vi "New Project.vi"(9 "DBSet":T1={"Server"="172.20.23.107", "DB"="HTPSDB", "PSW"="data'songyy", "User"="sa"}, 10 "UserID":string="L043460", 11 "厂区":string="清溪") -> ()   [LabVIEW 2011] (continued)
\n7714787500.000000#-39.000000#-4.400000#-18.000000#-10.000000#-3.000000#-30.000000#-30.000000\r\n7721031250.000000#-39.000000#-4.400000#-18.000000#-10.000000#-3.000000#-30.000000#-30.000000\r\n7727275000.000000#-39.000000#-4.400000#-18.000000#-10.000000#-3.000000#-30.000000#-30.000000\r\n7733518750.000000#-39.000000#-4.400000#-18.000000#-10.000000#-3.000000#-30.000000#-30.000000\r\n7739762500.000000#-39.000000#-4.400000#-18.000000#-10.000000#-3.000000#-30.000000#-30.000000\r\n7746006250.000000#-39.000000#-4.400000#-18.000000#-10.000000#-3.000000#-30.000000#-30.000000\r\n7752250000.000000#-39.000000#-4.400000#-18.000000#-10.000000#-3.000000#-30.000000#-30.000000\r\n7758493750.000000#-39.000000#-4.400000#-18.000000#-10.000000#-3.000000#-30.000000#-30.000000\r\n7764737500.000000#-39.000000#-4.400000#-18.000000#-10.000000#-3.000000#-30.000000#-30.000000\r\n7770981250.000000#-39.000000#-4.400000#-18.000000#-10.000000#-3.000000#-30.000000#-30.000000\r\n7777225000.000000#-39.000000#-4.400000#-18.000000#-10.000000#-3.000000#-30.000000#-30.000000\r\n7783468750.000000#-39.000000#-4.400000#-18.000000#-10.000000#-3.000000#-30.000000#-30.000000\r\n7789712500.000000#-39.000000#-4.400000#-18.000000#-10.000000#-3.000000#-30.000000#-30.000000\r\n7795956250.000000#-39.000000#-4.400000#-18.000000#-10.000000#-3.000000#-30.000000#-30.000000\r\n7802200000.000000#-39.000000#-4.400000#-18.000000#-10.000000#-3.000000#-30.000000#-30.000000\r\n7808443750.000000#-39.000000#-4.400000#-18.000000#-10.000000#-3.000000#-30.000000#-30.000000\r\n7814687500.000000#-39.000000#-4.400000#-18.000000#-10.000000#-3.000000#-30.000000#-30.000000\r\n7820931250.000000#-39.000000#-4.400000#-18.000000#-10.000000#-3.000000#-30.000000#-30.000000\r\n7827175000.000000#-39.000000#-4.400000#-18.000000#-10.000000#-3.000000#-30.000000#-30.000000\r\n7833418750.000000#-39.000000#-4.400000#-18.000000#-10.000000#-3.000000#-30.000000#-30.000000\r\n7839662500.000000#-39.000000#-4.400000#-18.000000#-10.000000#-3.000000#-30.000000#-30.000000\r\n7845906250.000000#-39.000000#-4.400000#-18.000000#-10.000000#-3.000000#-30.000000#-30.000000\r\n7852150000.000000#-39.000000#-4.400000#-18.000000#-10.000000#-3.000000#-30.000000#-30.000000\r\n7858393750.000000#-39.000000#-4.400000#-18.000000#-10.000000#-3.000000#-30.000000#-30.000000\r\n7864637500.000000#-39.000000#-4.400000#-18.000000#-10.000000#-3.000000#-30.000000#-30.000000\r\n7870881250.000000#-39.000000#-4.400000#-18.000000#-10.000000#-3.000000#-30.000000#-30.000000\r\n7877125000.000000#-39.000000#-4.400000#-18.000000#-10.000000#-3.000000#-30.000000#-30.000000\r\n7883368750.000000#-39.000000#-4.400000#-18.000000#-10.000000#-3.000000#-30.000000#-30.000000\r\n7889612500.000000#-39.000000#-4.400000#-18.000000#-10.000000#-3.000000#-30.000000#-30.000000\r\n7895856250.000000#-39.000000#-4.400000#-18.000000#-10.000000#-3.000000#-30.000000#-30.000000\r\n7902100000.000000#-39.000000#-4.400000#-18.000000#-10.000000#-3.000000#-30.000000#-30.000000\r\n7908343750.000000#-39.000000#-4.400000#-18.000000#-10.000000#-3.000000#-30.000000#-30.000000\r\n7914587500.000000#-39.000000#-4.400000#-18.000000#-10.000000#-3.000000#-30.000000#-30.000000\r\n7920831250.000000#-39.000000#-4.400000#-18.000000#-10.000000#-3.000000#-30.000000#-30.000000\r\n7927075000.000000#-39.000000#-4.400000#-18.000000#-10.000000#-3.000000#-30.000000#-30.000000\r\n7933318750.000000#-39.000000#-4.400000#-18.000000#-10.000000#-3.000000#-30.000000#-30.000000\r\n7939562500.000000#-39.000000#-4.400000#-18.000000#-10.000000#-3.000000#-30.000000#-30.000000\r\n7945806250.000000#-39.000000#-4.400000#-18.000000#-10.000000#-3.000000#-30.000000#-30.000000\r\n7952050000.000000#-39.000000#-4.400000#-18.000000#-10.000000#-3.000000#-30.000000#-30.000000\r\n7958293750.000000#-39.000000#-4.400000#-18.000000#-10.000000#-3.000000#-30.000000#-30.000000\r\n7964537500.000000#-39.000000#-4.400000#-18.000000#-10.000000#-3.000000#-30.000000#-30.000000\r\n7970781250.000000#-39.000000#-4.400000#-18.000000#-10.000000#-3.000000#-30.000000#-30.000000\r\n7977025000.000000#-39.000000#-4.400000#-18.000000#-10.000000#-3.000000#-30.000000#-30.000000\r\n7983268750.000000#-39.000000#-4.400000#-18.000000#-10.000000#-3.000000#-30.000000#-30.000000\r\n7989512500.000000#-39.000000#-4.400000#-18.000000#-10.000000#-3.000000#-30.000000#-30.000000\r\n7995756250.000000#-39.000000#-4.400000#-18.000000#-10.000000#-3.000000#-30.000000#-30.000000\r\n8002000000.000000#-39.000000#-4.400000#-18.000000#-10.000000#-3.000000#-30.000000#-30.000000\r\n8008243750.000000#-39.000000#-4.400000#-18.000000#-10.000000#-3.000000#-30.000000#-30.000000\r\n8014487500.000000#-39.000000#-4.400000#-18.000000#-10.000000#-3.000000#-30.000000#-30.000000\r\n8020731250.000000#-39.000000#-4.400000#-18.000000#-10.000000#-3.000000#-30.000000#-30.000000\r\n8026975000.000000#-39.000000#-4.400000#-18.000000#-10.000000#-3.000000#-30.000000#-30.000000\r\n8033218750.000000#-39.000000#-4.400000#-18.000000#-10.000000#-3.000000#-30.000000#-30.000000\r\n8039462500.000000#-39.000000#-4.400000#-18.000000#-10.000000#-3.000000#-30.000000#-30.000000\r\n8045706250.000000#-39.000000#-4.400000#-18.000000#-10.000000#-3.000000#-30.000000#-30.000000\r\n8051950000.000000#-39.000000#-4.400000#-18.000000#-10.000000#-3.000000#-30.000000#-30.000000\r\n8058193750.000000#-39.000000#-4.400000#-18.000000#-10.000000#-3.000000#-30.000000#-30.000000\r\n8064437500.000000#-39.000000#-4.400000#-18.000000#-10.000000#-3.000000#-30.000000#-30.000000\r\n8070681250.000000#-39.000000#-4.400000#-18.000000#-10.000000#-3.000000#-30.000000#-30.000000\r\n8076925000.000000#-39.000000#-4.400000#-18.000000#-10.000000#-3.000000#-30.000000#-30.000000\r\n8083168750.000000#-39.000000#-4.400000#-18.000000#-10.000000#-3.000000#-30.000000#-30.000000\r\n8089412500.000000#-39.000000#-4.400000#-18.000000#-10.000000#-3.000000#-30.000000#-30.000000\r\n8095656250.000000#-39.000000#-4.400000#-18.000000#-10.000000#-3.000000#-30.000000#-30.000000\r\n8101900000.000000#-39.000000#-4.400000#-18.000000#-10.000000#-3.000000#-30.000000#-30.000000\r\n8108143750.000000#-39.000000#-4.400000#-18.000000#-10.000000#-3.000000#-30.000000#-30.000000\r\n8114387500.000000#-39.000000#-4.400000#-18.000000#-10.000000#-3.000000#-30.000000#-30.000000\r\n8120631250.000000#-39.000000#-4.400000#-18.000000#-10.000000#-3.000000#-30.000000#-30.000000\r\n8126875000.000000#-39.000000#-4.400000#-18.000000#-10.000000#-3.000000#-30.000000#-30.000000\r\n8133118750.000000#-39.000000#-4.400000#-18.000000#-10.000000#-3.000000#-30.000000#-30.000000\r\n8139362500.000000#-39.000000#-4.400000#-18.000000#-10.000000#-3.000000#-30.000000#-30.000000\r\n8145606250.000000#-39.000000#-4.400000#-18.000000#-10.000000#-3.000000#-30.000000#-30.000000\r\n8151850000.000000#-39.000000#-4.400000#-18.000000#-10.000000#-3.000000#-30.000000#-30.000000\r\n8158093750.000000#-39.000000#-4.400000#-18.000000#-10.000000#-3.000000#-30.000000#-30.000000\r\n8164337500.000000#-39.000000#-4.400000#-18.000000#-10.000000#-3.000000#-30.000000#-30.000000\r\n8170581250.000000#-39.000000#-4.400000#-18.000000#-10.000000#-3.000000#-30.000000#-30.000000\r\n8176825000.000000#-39.000000#-4.400000#-18.000000#-10.000000#-3.000000#-30.000000#-30.000000\r\n8183068750.000000#-39.000000#-4.400000#-18.000000#-10.000000#-3.000000#-30.000000#-30.000000\r\n8189312500.000000#-39.000000#-4.400000#-18.000000#-10.000000#-3.000000#-30.000000#-30.000000\r\n8195556250.000000#-39.000000#-4.400000#-18.000000#-10.000000#-3.000000#-30.000000#-30.000000\r\n8201800000.000000#-39.000000#-4.400000#-18.000000#-10.000000#-3.000000#-30.000000#-30.000000\r\n8208043750.000000#-39.000000#-4.400000#-18.000000#-10.000000#-3.000000#-30.000000#-30.000000\r\n8214287500.000000#-39.000000#-4.400000#-18.000000#-10.000000#-3.000000#-30.000000#-30.000000\r\n8220531250.000000#-39.000000#-4.400000#-18.000000#-10.000000#-3.000000#-30.000000#-30.000000\r\n8226775000.000000#-39.000000#-4.400000#-18.000000#-10.000000#-3.000000#-30.000000#-30.000000\r\n8233018750.000000#-39.000000#-4.400000#-18.000000#-10.000000#-3.000000#-30.000000#-30.000000\r\n8239262500.000000#-39.000000#-4.400000#-18.000000#-10.000000#-3.000000#-30.000000#-30.000000\r\n8245506250.000000#-39.000000#-4.400000#-18.000000#-10.000000#-3.000000#-30.000000#-30.000000\r\n8251750000.000000#-39.000000#-4.400000#-18.000000#-10.000000#-3.000000#-30.000000#-30.000000\r\n8257993750.000000#-39.000000#-4.400000#-18.000000#-10.000000#-3.000000#-30.000000#-30.000000\r\n8264237500.000000#-39.000000#-4.400000#-18.000000#-10.000000#-3.000000#-30.000000#-30.000000\r\n8270481250.000000#-39.000000#-4.400000#-18.000000#-10.000000#-3.000000#-30.000000#-30.000000\r\n8276725000.000000#-39.000000#-4.400000#-18.000000#-10.000000#-3.000000#-30.000000#-30.000000\r\n8282968750.000000#-39.000000#-4.400000#-18.000000#-10.000000#-3.000000#-30.000000#-30.000000\r\n8289212500.000000#-39.000000#-4.400000#-18.000000#-10.000000#-3.000000#-30.000000#-30.000000\r\n8295456250.000000#-39.000000#-4.400000#-18.000000#-10.000000#-3.000000#-30.000000#-30.000000\r\n8301700000.000000#-39.000000#-4.400000#-18.000000#-10.000000#-3.000000#-30.000000#-30.000000\r\n8307943750.000000#-39.000000#-4.400000#-18.000000#-10.000000#-3.000000#-30.000000#-30.000000\r\n8314187500.000000#-39.000000#-4.400000#-18.000000#-10.000000#-3.000000#-30.000000#-30.000000\r\n8320431250.000000#-39.000000#-4.400000#-18.000000#-10.000000#-3.000000#-30.000000#-30.000000\r\n8326675000.000000#-39.000000#-4.400000#-18.000000#-10.000000#-3.000000#-30.000000#-30.000000\r\n8332918750.000000#-39.000000#-4.400000#-18.000000#-10.000000#-3.000000#-30.000000#-30.000000\r\n8339162500.000000#-39.000000#-4.400000#-18.000000#-10.000000#-3.000000#-30.000000#-30.000000\r\n8345406250.000000#-39.000000#-4.400000#-18.000000#-10.000000#-3.000000#-30.000000#-30.000000\r\n8351650000.000000#-39.000000#-4.400000#-18.000000#-10.000000#-3.000000#-30.000000#-30.000000\r\n8357893750.000000#-39.000000#-4.400000#-18.000000#-10.000000#-3.000000#-30.000000#-30.000000\r\n8364137500.000000#-39.000000#-4.400000#-18.000000#-10.000000#-3.000000#-30.000000#-30.000000\r\n8370381250.000000#-39.000000#-4.400000#-18.000000#-10.000000#-3.000000#-30.000000#-30.000000\r\n8376625000.000000#-39.000000#-4.400000#-18.000000#-10.000000#-3.000000#-30.000000#-30.000000\r\n8382868750.000000#-39.000000#-4.400000#-18.000000#-10.000000#-3.000000#-30.000000#-30.000000\r\n8389112500.000000#-39.000000#-4.400000#-18.000000#-10.000000#-3.000000#-30.000000#-30.000000\r\n8395356250.000000#-39.000000#-4.400000#-18.000000#-10.000000#-3.000000#-30.000000#-30.000000\r\n8401600000.000000#-39.000000#-4.400000#-18.000000#-10.000000#-3.000000#-30.000000#-30.000000\r\n8407843750.000000#-39.000000#-4.400000#-18.000000#-10.000000#-3.000000#-30.000000#-30.000000\r\n8414087500.000000#-39.000000#-4.400000#-18.000000#-10.000000#-3.000000#-30.000000#-30.000000\r\n8420331250.000000#-39.000000#-4.400000#-18.000000#-10.000000#-3.000000#-30.000000#-30.000000\r\n8426575000.000000#-39.000000#-4.400000#-18.000000#-10.000000#-3.000000#-30.000000#-30.000000\r\n8432818750.000000#-39.000000#-4.400000#-18.000000#-10.000000#-3.000000#-30.000000#-30.000000\r\n8439062500.000000#-39.000000#-4.400000#-18.000000#-10.000000#-3.000000#-30.000000#-30.000000\r\n8445306250.000000#-39.000000#-4.400000#-18.000000#-10.000000#-3.000000#-30.000000#-30.000000\r\n8451550000.000000#-39.000000#-4.400000#-18.000000#-10.000000#-3.000000#-30.000000#-30.000000\r\n8457793750.000000#-39.000000#-4.400000#-18.000000#-10.000000#-3.000000#-30.000000#-30.000000\r\n8464037500.000000#-39.000000#-4.400000#-18.000000#-10.000000#-3.000000#-30.000000#-30.000000\r\n8470281250.000000#-39.000000#-4.400000#-18.000000#-10.000000#-3.000000#-30.000000#-30.000000\r\n8476525000.000000#-39.000000#-4.400000#-18.000000#-10.000000#-3.000000#-30.000000#-30.000000\r\n8482768750.000000#-39.000000#-4.400000#-18.000000#-10.000000#-3.000000#-30.000000#-30.000000\r\n8489012500.000000#-39.000000#-4.400000#-18.000000#-10.000000#-3.000000#-30.000000#-30.000000\r\n8495256250.000000#-39.000000#-4.400000#-18.000000#-10.000000#-3.000000#-30.000000#-30.000000\r\n8501500000.000000#-39.000000#-4.400000#-18.000000#-10.000000#-3.000000#-30.000000#-30.000000\r\n8507743750.000000#-39.000000#-4.400000#-18.000000#-10.000000#-3.000000#-30.000000#-30.000000\r\n8513987500.000000#-39.000000#-4.400000#-18.000000#-10.000000#-3.000000#-30.000000#-30.000000\r\n8520231250.000000#-39.000000#-4.400000#-18.000000#-10.000000#-3.000000#-30.000000#-30.000000\r\n8526475000.000000#-39.000000#-4.400000#-18.000000#-10.000000#-3.000000#-30.000000#-30.000000\r\n8532718750.000000#-39.000000#-4.400000#-18.000000#-10.000000#-3.000000#-30.000000#-30.000000\r\n8538962500.000000#-39.000000#-4.400000#-18.000000#-10.000000#-3.000000#-30.000000#-30.000000\r\n8545206250.000000#-39.000000#-4.400000#-18.000000#-10.000000#-3.000000#-30.000000#-30.000000\r\n8551450000.000000#-39.000000#-4.400000#-18.000000#-10.000000#-3.000000#-30.000000#-30.000000\r\n8557693750.000000#-39.000000#-4.400000#-18.000000#-10.000000#-3.000000#-30.000000#-30.000000\r\n8563937500.000000#-39.000000#-4.400000#-18.000000#-10.000000#-3.000000#-30.000000#-30.000000\r\n8570181250.000000#-39.000000#-4.400000#-18.000000#-10.000000#-3.000000#-30.000000#-30.000000\r\n8576425000.000000#-39.000000#-4.400000#-18.000000#-10.000000#-3.000000#-30.000000#-30.000000\r\n8582668750.000000#-39.000000#-4.400000#-18.000000#-10.000000#-3.000000#-30.000000#-30.000000\r\n8588912500.000000#-39.000000#-4.400000#-18.000000#-10.000000#-3.000000#-30.000000#-30.000000\r\n8595156250.000000#-39.000000#-4.400000#-18.000000#-10.000000#-3.000000#-30.000000#-30.000000\r\n8601400000.000000#-39.000000#-4.400000#-18.000000#-10.000000#-3.000000#-30.000000#-30.000000\r\n8607643750.000000#-39.000000#-4.400000#-18.000000#-10.000000#-3.000000#-30.000000#-30.000000\r\n8613887500.000000#-39.000000#-4.400000#-18.000000#-10.000000#-3.000000#-30.000000#-30.000000\r\n8620131250.000000#-39.000000#-4.400000#-18.000000#-10.000000#-3.000000#-30.000000#-30.000000\r\n8626375000.000000#-39.000000#-4.400000#-18.000000#-10.000000#-3.000000#-30.000000#-30.000000\r\n8632618750.000000#-39.000000#-4.400000#-18.000000#-10.000000#-3.000000#-30.000000#-30.000000\r\n8638862500.000000#-39.000000#-4.400000#-18.000000#-10.000000#-3.000000#-30.000000#-30.000000\r\n8645106250.000000#-39.000000#-4.400000#-18.000000#-10.000000#-3.000000#-30.000000#-30.000000\r\n8651350000.000000#-39.000000#-4.400000#-18.000000#-10.000000#-3.000000#-30.000000#-30.000000\r\n8657593750.000000#-39.000000#-4.400000#-18.000000#-10.000000#-3.000000#-30.000000#-30.000000\r\n8663837500.000000#-39.000000#-4.400000#-18.000000#-10.000000#-3.000000#-30.000000#-30.000000\r\n8670081250.000000#-39.000000#-4.400000#-18.000000#-10.000000#-3.000000#-30.000000#-30.000000\r\n8676325000.000000#-39.000000#-4.400000#-18.000000#-10.000000#-3.000000#-30.000000#-30.000000\r\n8682568750.000000#-39.000000#-4.400000#-18.000000#-10.000000#-3.000000#-30.000000#-30.000000\r\n8688812500.000000#-39.000000#-4.400000#-18.000000#-10.000000#-3.000000#-30.000000#-30.000000\r\n8695056250.000000#-39.000000#-4.400000#-18.000000#-10.000000#-3.000000#-30.000000#-30.000000\r\n8701300000.000000#-39.000000#-4.400000#-18.000000#-10.000000#-3.000000#-30.000000#-30.000000\r\n8707543750.000000#-39.000000#-4.400000#-18.000000#-10.000000#-3.000000#-30.000000#-30.000000\r\n8713787500.000000#-39.000000#-4.400000#-18.000000#-10.000000#-3.000000#-30.000000#-30.000000\r\n8720031250.000000#-39.000000#-4.400000#-18.000000#-10.000000#-3.000000#-30.000000#-30.000000\r\n8726275000.000000#-39.000000#-4.400000#-18.000000#-10.000000#-3.000000#-30.000000#-30.000000\r\n8732518750.000000#-39.000000#-4.400000#-18.000000#-10.000000#-3.000000#-30.000000#-30.000000\r\n8738762500.000000#-39.000000#-4.400000#-18.000000#-10.000000#-3.000000#-30.000000#-30.000000\r\n8745006250.000000#-39.000000#-4.400000#-18.000000#-10.000000#-3.000000#-30.000000#-30.000000\r\n8751250000.000000#-39.000000#-4.400000#-18.000000#-10.000000#-3.000000#-30.000000#-30.000000\r\n8757493750.000000#-39.000000#-4.400000#-18.000000#-10.000000#-3.000000#-30.000000#-30.000000\r\n8763737500.000000#-39.000000#-4.400000#-18.000000#-10.000000#-3.000000#-30.000000#-30.000000\r\n8769981250.000000#-39.000000#-4.400000#-18.000000#-10.000000#-3.000000#-30.000000#-30.000000\r\n8776225000.000000#-39.000000#-4.400000#-18.000000#-10.000000#-3.000000#-30.000000#-30.000000\r\n8782468750.000000#-39.000000#-4.400000#-18.000000#-10.000000#-3.000000#-30.000000#-30.000000\r\n8788712500.000000#-39.000000#-4.400000#-18.000000#-10.000000#-3.000000#-30.000000#-30.000000\r\n8794956250.000000#-39.000000#-4.400000#-18.000000#-10.000000#-3.000000#-30.000000#-30.000000\r\n8801200000.000000#-39.000000#-4.400000#-18.000000#-10.000000#-3.000000#-30.000000#-30.000000\r\n8807443750.000000#-39.000000#-4.400000#-18.000000#-10.000000#-3.000000#-30.000000#-30.000000\r\n8813687500.000000#-39.000000#-4.400000#-18.000000#-10.000000#-3.000000#-30.000000#-30.000000\r\n8819931250.000000#-39.000000#-4.400000#-18.000000#-10.000000#-3.000000#-30.000000#-30.000000\r\n8826175000.000000#-39.000000#-4.400000#-18.000000#-10.000000#-3.000000#-30.000000#-30.000000\r\n8832418750.000000#-39.000000#-4.400000#-18.000000#-10.000000#-3.000000#-30.000000#-30.000000\r\n8838662500.000000#-39.000000#-4.400000#-18.000000#-10.000000#-3.000000#-30.000000#-30.000000\r\n8844906250.000000#-39.000000#-4.400000#-18.000000#-10.000000#-3.000000#-30.000000#-30.000000\r\n8851150000.000000#-39.000000#-4.400000#-18.000000#-10.000000#-3.000000#-30.000000#-30.000000\r\n8857393750.000000#-39.000000#-4.400000#-18.000000#-10.000000#-3.000000#-30.000000#-30.000000\r\n8863637500.000000#-39.000000#-4.400000#-18.000000#-10.000000#-3.000000#-30.000000#-30.000000\r\n8869881250.000000#-39.000000#-4.400000#-18.000000#-10.000000#-3.000000#-30.000000#-30.000000\r\n8876125000.000000#-39.000000#-4.400000#-18.000000#-10.000000#-3.000000#-30.000000#-30.000000\r\n8882368750.000000#-39.000000#-4.400000#-18.000000#-10.000000#-3.000000#-30.000000#-30.000000\r\n8888612500.000000#-39.000000#-4.400000#-18.000000#-10.000000#-3.000000#-30.000000#-30.000000\r\n8894856250.000000#-39.000000#-4.400000#-18.000000#-10.000000#-3.000000#-30.000000#-30.000000\r\n8901100000.000000#-39.000000#-4.400000#-18.000000#-10.000000#-3.000000#-30.000000#-30.000000\r\n8907343750.000000#-39.000000#-4.400000#-18.000000#-10.000000#-3.000000#-30.000000#-30.000000\r\n8913587500.000000#-39.000000#-4.400000#-18.000000#-10.000000#-3.000000#-30.000000#-30.000000\r\n8919831250.000000#-39.000000#-4.400000#-18.000000#-10.000000#-3.000000#-30.000000#-30.000000\r\n8926075000.000000#-39.000000#-4.400000#-18.000000#-10.000000#-3.000000#-30.000000#-30.000000\r\n8932318750.000000#-39.000000#-4.400000#-18.000000#-10.000000#-3.000000#-30.000000#-30.000000\r\n8938562500.000000#-39.000000#-4.400000#-18.000000#-10.000000#-3.000000#-30.000000#-30.000000\r\n8944806250.000000#-39.000000#-4.400000#-18.000000#-10.000000#-3.000000#-30.000000#-30.000000\r\n8951050000.000000#-39.000000#-4.400000#-18.000000#-10.000000#-3.000000#-30.000000#-30.000000\r\n8957293750.000000#-39.000000#-4.400000#-18.000000#-10.000000#-3.000000#-30.000000#-30.000000\r\n8963537500.000000#-39.000000#-4.400000#-18.000000#-10.000000#-3.000000#-30.000000#-30.000000\r\n8969781250.000000#-39.000000#-4.400000#-18.000000#-10.000000#-3.000000#-30.000000#-30.000000\r\n8976025000.000000#-39.000000#-4.400000#-18.000000#-10.000000#-3.000000#-30.000000#-30.000000\r\n8982268750.000000#-39.000000#-4.400000#-18.000000#-10.000000#-3.000000#-30.000000#-30.000000\r\n8988512500.000000#-39.000000#-4.400000#-18.000000#-10.000000#-3.000000#-30.000000#-30.000000\r\n8994756250.000000#-39.000000#-4.400000#-18.000000#-10.000000#-3.000000#-30.000000#-30.000000\r\n9001000000.000000#-39.000000#-4.400000#-18.000000#-10.000000#-3.000000#-30.000000#-30.000000\r\n9007243750.000000#-39.000000#-3.500000#-18.000000#-10.000000#-3.000000#-30.000000#-30.000000\r\n9013487500.000000#-39.000000#-3.500000#-18.000000#-10.000000#-3.000000#-30.000000#-30.000000\r\n9019731250.000000#-39.000000#-3.500000#-18.000000#-10.000000#-3.000000#-30.000000#-30.000000\r\n9025975000.000000#-39.000000#-3.500000#-18.000000#-10.000000#-3.000000#-30.000000#-30.000000\r\n9032218750.000000#-39.000000#-3.500000#-18.000000#-10.000000#-3.000000#-30.000000#-30.000000\r\n9038462500.000000#-39.000000#-3.500000#-18.000000#-10.000000#-3.000000#-30.000000#-30.000000\r\n9044706250.000000#-39.000000#-3.500000#-18.000000#-10.000000#-3.000000#-30.000000#-30.000000\r\n9050950000.000000#-39.000000#-3.500000#-18.000000#-10.000000#-3.000000#-30.000000#-30.000000\r\n9057193750.000000#-39.000000#-3.500000#-18.000000#-10.000000#-3.000000#-30.000000#-30.000000\r\n9063437500.000000#-39.000000#-3.500000#-18.000000#-10.000000#-3.000000#-30.000000#-30.000000\r\n9069681250.000000#-39.000000#-3.500000#-18.000000#-10.000000#-3.000000#-30.000000#-30.000000\r\n9075925000.000000#-39.000000#-3.500000#-18.000000#-10.000000#-3.000000#-30.000000#-30.000000\r\n9082168750.000000#-39.000000#-3.500000#-18.000000#-10.000000#-3.000000#-30.000000#-30.000000\r\n9088412500.000000#-39.000000#-3.500000#-18.000000#-10.000000#-3.000000#-30.000000#-30.000000\r\n9094656250.000000#-39.000000#-3.500000#-18.000000#-10.000000#-3.000000#-30.000000#-30.000000\r\n9100900000.000000#-39.000000#-3.500000#-18.000000#-10.000000#-3.000000#-30.000000#-30.000000\r\n9107143750.000000#-39.000000#-3.500000#-18.000000#-10.000000#-3.000000#-30.000000#-30.000000\r\n9113387500.000000#-39.000000#-3.500000#-18.000000#-10.000000#-3.000000#-30.000000#-30.000000\r\n9119631250.000000#-39.000000#-3.500000#-18.000000#-10.000000#-3.000000#-30.000000#-30.000000\r\n9125875000.000000#-39.000000#-3.500000#-18.000000#-10.000000#-3.000000#-30.000000#-30.000000\r\n9132118750.000000#-39.000000#-3.500000#-18.000000#-10.000000#-3.000000#-30.000000#-30.000000\r\n9138362500.000000#-39.000000#-3.500000#-18.000000#-10.000000#-3.000000#-30.000000#-30.000000\r\n9144606250.000000#-39.000000#-3.500000#-18.000000#-10.000000#-3.000000#-30.000000#-30.000000\r\n9150850000.000000#-39.000000#-3.500000#-18.000000#-10.000000#-3.000000#-30.000000#-30.000000\r\n9157093750.000000#-39.000000#-3.500000#-18.000000#-10.000000#-3.000000#-30.000000#-30.000000\r\n9163337500.000000#-39.000000#-3.500000#-18.000000#-10.000000#-3.000000#-30.000000#-30.000000\r\n9169581250.000000#-39.000000#-3.500000#-18.000000#-10.000000#-3.000000#-30.000000#-30.000000\r\n9175825000.000000#-39.000000#-3.500000#-18.000000#-10.000000#-3.000000#-30.000000#-30.000000\r\n9182068750.000000#-39.000000#-3.500000#-18.000000#-10.000000#-3.000000#-30.000000#-30.000000\r\n9188312500.000000#-39.000000#-3.500000#-18.000000#-10.000000#-3.000000#-30.000000#-30.000000\r\n9194556250.000000#-39.000000#-3.500000#-18.000000#-10.000000#-3.000000#-30.000000#-30.000000\r\n9200800000.000000#-39.000000#-3.500000#-18.000000#-10.000000#-3.000000#-30.000000#-30.000000\r\n9207043750.000000#-39.000000#-3.500000#-18.000000#-10.000000#-3.000000#-30.000000#-30.000000\r\n9213287500.000000#-39.000000#-3.500000#-18.000000#-10.000000#-3.000000#-30.000000#-30.000000\r\n9219531250.000000#-39.000000#-3.500000#-18.000000#-10.000000#-3.000000#-30.000000#-30.000000\r\n9225775000.000000#-39.000000#-3.500000#-18.000000#-10.000000#-3.000000#-30.000000#-30.000000\r\n9232018750.000000#-39.000000#-3.500000#-18.000000#-10.000000#-3.000000#-30.000000#-30.000000\r\n9238262500.000000#-39.000000#-3.500000#-18.000000#-10.000000#-3.000000#-30.000000#-30.000000\r\n9244506250.000000#-39.000000#-3.500000#-18.000000#-10.000000#-3.000000#-30.000000#-30.000000\r\n9250750000.000000#-39.000000#-3.500000#-18.000000#-10.000000#-3.000000#-30.000000#-30.000000\r\n9256993750.000000#-39.000000#-3.500000#-18.000000#-10.000000#-3.000000#-30.000000#-30.000000\r\n9263237500.000000#-39.000000#-3.500000#-18.000000#-10.000000#-3.000000#-30.000000#-30.000000\r\n9269481250.000000#-39.000000#-3.500000#-18.000000#-10.000000#-3.000000#-30.000000#-30.000000\r\n9275725000.000000#-39.000000#-3.500000#-18.000000#-10.000000#-3.000000#-30.000000#-30.000000\r\n9281968750.000000#-39.000000#-3.500000#-18.000000#-10.000000#-3.000000#-30.000000#-30.000000\r\n9288212500.000000#-39.000000#-3.500000#-18.000000#-10.000000#-3.000000#-30.000000#-30.000000\r\n9294456250.000000#-39.000000#-3.500000#-18.000000#-10.000000#-3.000000#-30.000000#-30.000000\r\n9300700000.000000#-39.000000#-3.500000#-18.000000#-10.000000#-3.000000#-30.000000#-30.000000\r\n9306943750.000000#-39.000000#-3.500000#-18.000000#-10.000000#-3.000000#-30.000000#-30.000000\r\n9313187500.000000#-39.000000#-3.500000#-18.000000#-10.000000#-3.000000#-30.000000#-30.000000\r\n9319431250.000000#-39.000000#-3.500000#-18.000000#-10.000000#-3.000000#-30.000000#-30.000000\r\n9325675000.000000#-39.000000#-3.500000#-18.000000#-10.000000#-3.000000#-30.000000#-30.000000\r\n9331918750.000000#-39.000000#-3.500000#-18.000000#-10.000000#-3.000000#-30.000000#-30.000000\r\n9338162500.000000#-39.000000#-3.500000#-18.000000#-10.000000#-3.000000#-30.000000#-30.000000\r\n9344406250.000000#-39.000000#-3.500000#-18.000000#-10.000000#-3.000000#-30.000000#-30.000000\r\n9350650000.000000#-39.000000#-3.500000#-18.000000#-10.000000#-3.000000#-30.000000#-30.000000\r\n9356893750.000000#-39.000000#-3.500000#-18.000000#-10.000000#-3.000000#-30.000000#-30.000000\r\n9363137500.000000#-39.000000#-3.500000#-18.000000#-10.000000#-3.000000#-30.000000#-30.000000\r\n9369381250.000000#-39.000000#-3.500000#-18.000000#-10.000000#-3.000000#-30.000000#-30.000000\r\n9375625000.000000#-39.000000#-3.500000#-18.000000#-10.000000#-3.000000#-30.000000#-30.000000\r\n9381868750.000000#-39.000000#-3.500000#-18.000000#-10.000000#-3.000000#-30.000000#-30.000000\r\n9388112500.000000#-39.000000#-3.500000#-18.000000#-10.000000#-3.000000#-30.000000#-30.000000\r\n9394356250.000000#-39.000000#-3.500000#-18.000000#-10.000000#-3.000000#-30.000000#-30.000000\r\n9400600000.000000#-39.000000#-3.500000#-18.000000#-10.000000#-3.000000#-30.000000#-30.000000\r\n9406843750.000000#-39.000000#-3.500000#-18.000000#-10.000000#-3.000000#-30.000000#-30.000000\r\n9413087500.000000#-39.000000#-3.500000#-18.000000#-10.000000#-3.000000#-30.000000#-30.000000\r\n9419331250.000000#-39.000000#-3.500000#-18.000000#-10.000000#-3.000000#-30.000000#-30.000000\r\n9425575000.000000#-39.000000#-3.500000#-18.000000#-10.000000#-3.000000#-30.000000#-30.000000\r\n9431818750.000000#-39.000000#-3.500000#-18.000000#-10.000000#-3.000000#-30.000000#-30.000000\r\n9438062500.000000#-39.000000#-3.500000#-18.000000#-10.000000#-3.000000#-30.000000#-30.000000\r\n9444306250.000000#-39.000000#-3.500000#-18.000000#-10.000000#-3.000000#-30.000000#-30.000000\r\n9450550000.000000#-39.000000#-3.500000#-18.000000#-10.000000#-3.000000#-30.000000#-30.000000\r\n9456793750.000000#-39.000000#-3.500000#-18.000000#-10.000000#-3.000000#-30.000000#-30.000000\r\n9463037500.000000#-39.000000#-3.500000#-18.000000#-10.000000#-3.000000#-30.000000#-30.000000\r\n9469281250.000000#-39.000000#-3.500000#-18.000000#-10.000000#-3.000000#-30.000000#-30.000000\r\n9475525000.000000#-39.000000#-3.500000#-18.000000#-10.000000#-3.000000#-30.000000#-30.000000\r\n9481768750.000000#-39.000000#-3.500000#-18.000000#-10.000000#-3.000000#-30.000000#-30.000000\r\n9488012500.000000#-39.000000#-3.500000#-18.000000#-10.000000#-3.000000#-30.000000#-30.000000\r\n9494256250.000000#-39.000000#-3.500000#-18.000000#-10.000000#-3.000000#-30.000000#-30.000000\r\n9500500000.000000#-39.000000#-3.500000#-18.000000#-10.000000#-3.000000#-30.000000#-30.000000\r\n9506743750.000000#-39.000000#-3.500000#-18.000000#-10.000000#-3.000000#-30.000000#-30.000000\r\n9512987500.000000#-39.000000#-3.500000#-18.000000#-10.000000#-3.000000#-30.000000#-30.000000\r\n9519231250.000000#-39.000000#-3.500000#-18.000000#-10.000000#-3.000000#-30.000000#-30.000000\r\n9525475000.000000#-39.000000#-3.500000#-18.000000#-10.000000#-3.000000#-30.000000#-30.000000\r\n9531718750.000000#-39.000000#-3.500000#-18.000000#-10.000000#-3.000000#-30.000000#-30.000000\r\n9537962500.000000#-39.000000#-3.500000#-18.000000#-10.000000#-3.000000#-30.000000#-30.000000\r\n9544206250.000000#-39.000000#-3.500000#-18.000000#-10.000000#-3.000000#-30.000000#-30.000000\r\n9550450000.000000#-39.000000#-3.500000#-18.000000#-10.000000#-3.000000#-30.000000#-30.000000\r\n9556693750.000000#-39.000000#-3.500000#-18.000000#-10.000000#-3.000000#-30.000000#-30.000000\r\n9562937500.000000#-39.000000#-3.500000#-18.000000#-10.000000#-3.000000#-30.000000#-30.000000\r\n9569181250.000000#-39.000000#-3.500000#-18.000000#-10.000000#-3.000000#-30.000000#-30.000000\r\n9575425000.000000#-39.000000#-3.500000#-18.000000#-10.000000#-3.000000#-30.000000#-30.000000\r\n9581668750.000000#-39.000000#-3.500000#-18.000000#-10.000000#-3.000000#-30.000000#-30.000000\r\n9587912500.000000#-39.000000#-3.500000#-18.000000#-10.000000#-3.000000#-30.000000#-30.000000\r\n9594156250.000000#-39.000000#-3.500000#-18.000000#-10.000000#-3.000000#-30.000000#-30.000000\r\n9600400000.000000#-39.000000#-3.500000#-18.000000#-10.000000#-3.000000#-30.000000#-30.000000\r\n9606643750.000000#-39.000000#-3.500000#-18.000000#-10.000000#-3.000000#-30.000000#-30.000000\r\n9612887500.000000#-39.000000#-3.500000#-18.000000#-10.000000#-3.000000#-30.000000#-30.000000\r\n9619131250.000000#-39.000000#-3.500000#-18.000000#-10.000000#-3.000000#-30.000000#-30.000000\r\n9625375000.000000#-39.000000#-3.500000#-18.000000#-10.000000#-3.000000#-30.000000#-30.000000\r\n9631618750.000000#-39.000000#-3.500000#-18.000000#-10.000000#-3.000000#-30.000000#-30.000000\r\n9637862500.000000#-39.000000#-3.500000#-18.000000#-10.000000#-3.000000#-30.000000#-30.000000\r\n9644106250.000000#-39.000000#-3.500000#-18.000000#-10.000000#-3.000000#-30.000000#-30.000000\r\n9650350000.000000#-39.000000#-3.500000#-18.000000#-10.000000#-3.000000#-30.000000#-30.000000\r\n9656593750.000000#-39.000000#-3.500000#-18.000000#-10.000000#-3.000000#-30.000000#-30.000000\r\n9662837500.000000#-39.000000#-3.500000#-18.000000#-10.000000#-3.000000#-30.000000#-30.000000\r\n9669081250.000000#-39.000000#-3.500000#-18.000000#-10.000000#-3.000000#-30.000000#-30.000000\r\n9675325000.000000#-39.000000#-3.500000#-18.000000#-10.000000#-3.000000#-30.000000#-30.000000\r\n9681568750.000000#-39.000000#-3.500000#-18.000000#-10.000000#-3.000000#-30.000000#-30.000000\r\n9687812500.000000#-39.000000#-3.500000#-18.000000#-10.000000#-3.000000#-30.000000#-30.000000\r\n9694056250.000000#-39.000000#-3.500000#-18.000000#-10.000000#-3.000000#-30.000000#-30.000000\r\n9700300000.000000#-39.000000#-3.500000#-18.000000#-10.000000#-3.000000#-30.000000#-30.000000\r\n9706543750.000000#-39.000000#-3.500000#-18.000000#-10.000000#-3.000000#-30.000000#-30.000000\r\n9712787500.000000#-39.000000#-3.500000#-18.000000#-10.000000#-3.000000#-30.000000#-30.000000\r\n9719031250.000000#-39.000000#-3.500000#-18.000000#-10.000000#-3.000000#-30.000000#-30.000000\r\n9725275000.000000#-39.000000#-3.500000#-18.000000#-10.000000#-3.000000#-30.000000#-30.000000\r\n9731518750.000000#-39.000000#-3.500000#-18.000000#-10.000000#-3.000000#-30.000000#-30.000000\r\n9737762500.000000#-39.000000#-3.500000#-18.000000#-10.000000#-3.000000#-30.000000#-30.000000\r\n9744006250.000000#-39.000000#-3.500000#-18.000000#-10.000000#-3.000000#-30.000000#-30.000000\r\n9750250000.000000#-39.000000#-3.500000#-18.000000#-10.000000#-3.000000#-30.000000#-30.000000\r\n9756493750.000000#-39.000000#-3.500000#-18.000000#-10.000000#-3.000000#-30.000000#-30.000000\r\n9762737500.000000#-39.000000#-3.500000#-18.000000#-10.000000#-3.000000#-30.000000#-30.000000\r\n9768981250.000000#-39.000000#-3.500000#-18.000000#-10.000000#-3.000000#-30.000000#-30.000000\r\n9775225000.000000#-39.000000#-3.500000#-18.000000#-10.000000#-3.000000#-30.000000#-30.000000\r\n9781468750.000000#-39.000000#-3.500000#-18.000000#-10.000000#-3.000000#-30.000000#-30.000000\r\n9787712500.000000#-39.000000#-3.500000#-18.000000#-10.000000#-3.000000#-30.000000#-30.000000\r\n9793956250.000000#-39.000000#-3.500000#-18.000000#-10.000000#-3.000000#-30.000000#-30.000000\r\n9800200000.000000#-39.000000#-3.500000#-18.000000#-10.000000#-3.000000#-30.000000#-30.000000\r\n9806443750.000000#-39.000000#-3.500000#-18.000000#-10.000000#-3.000000#-30.000000#-30.000000\r\n9812687500.000000#-39.000000#-3.500000#-18.000000#-10.000000#-3.000000#-30.000000#-30.000000\r\n9818931250.000000#-39.000000#-3.500000#-18.000000#-10.000000#-3.000000#-30.000000#-30.000000\r\n9825175000.000000#-39.000000#-3.500000#-18.000000#-10.000000#-3.000000#-30.000000#-30.000000\r\n9831418750.000000#-39.000000#-3.500000#-18.000000#-10.000000#-3.000000#-30.000000#-30.000000\r\n9837662500.000000#-39.000000#-3.500000#-18.000000#-10.000000#-3.000000#-30.000000#-30.000000\r\n9843906250.000000#-39.000000#-3.500000#-18.000000#-10.000000#-3.000000#-30.000000#-30.000000\r\n9850150000.000000#-39.000000#-3.500000#-18.000000#-10.000000#-3.000000#-30.000000#-30.000000\r\n9856393750.000000#-39.000000#-3.500000#-18.000000#-10.000000#-3.000000#-30.000000#-30.000000\r\n9862637500.000000#-39.000000#-3.500000#-18.000000#-10.000000#-3.000000#-30.000000#-30.000000\r\n9868881250.000000#-39.000000#-3.500000#-18.000000#-10.000000#-3.000000#-30.000000#-30.000000\r\n9875125000.000000#-39.000000#-3.500000#-18.000000#-10.000000#-3.000000#-30.000000#-30.000000\r\n9881368750.000000#-39.000000#-3.500000#-18.000000#-10.000000#-3.000000#-30.000000#-30.000000\r\n9887612500.000000#-39.000000#-3.500000#-18.000000#-10.000000#-3.000000#-30.000000#-30.000000\r\n9893856250.000000#-39.000000#-3.500000#-18.000000#-10.000000#-3.000000#-30.000000#-30.000000\r\n9900100000.000000#-39.000000#-3.500000#-18.000000#-10.000000#-3.000000#-30.000000#-30.000000\r\n9906343750.000000#-39.000000#-3.500000#-18.000000#-10.000000#-3.000000#-30.000000#-30.000000\r\n9912587500.000000#-39.000000#-3.500000#-18.000000#-10.000000#-3.000000#-30.000000#-30.000000\r\n9918831250.000000#-39.000000#-3.500000#-18.000000#-10.000000#-3.000000#-30.000000#-30.000000\r\n9925075000.000000#-39.000000#-3.500000#-18.000000#-10.000000#-3.000000#-30.000000#-30.000000\r\n9931318750.000000#-39.000000#-3.500000#-18.000000#-10.000000#-3.000000#-30.000000#-30.000000\r\n9937562500.000000#-39.000000#-3.500000#-18.000000#-10.000000#-3.000000#-30.000000#-30.000000\r\n9943806250.000000#-39.000000#-3.500000#-18.000000#-10.000000#-3.000000#-30.000000#-30.000000\r\n9950050000.000000#-39.000000#-3.500000#-18.000000#-10.000000#-3.000000#-30.000000#-30.000000\r\n9956293750.000000#-39.000000#-3.500000#-18.000000#-10.000000#-3.000000#-30.000000#-30.000000\r\n9962537500.000000#-39.000000#-3.500000#-18.000000#-10.000000#-3.000000#-30.000000#-30.000000\r\n9968781250.000000#-39.000000#-3.500000#-18.000000#-10.000000#-3.000000#-30.000000#-30.000000\r\n9975025000.000000#-39.000000#-3.500000#-18.000000#-10.000000#-3.000000#-30.000000#-30.000000\r\n9981268750.000000#-39.000000#-3.500000#-18.000000#-10.000000#-3.000000#-30.000000#-30.000000\r\n9987512500.000000#-39.000000#-3.500000#-18.000000#-10.000000#-3.000000#-30.000000#-30.000000\r\n9993756250.000000#-39.000000#-3.500000#-18.000000#-10.000000#-3.000000#-30.000000#-30.000000\r\nNaN#NaN#NaN#NaN#NaN#NaN#NaN#NaN\r\n", "0#0#0#0#0#0#0#0#0#0#0#0#0#0#0#0#0#0#0#0#0#0#0#0#0#0#0#0#0#0#0#0#0#1#0#1#0#1#0#1#0#0#0#0#0#0#0#0#0#0#0#0#0#0#0#0#0#0#0#0#0#0#0#0#0#0#0#0#0#0#0#0#0#0#0#0#0#0#0#0#0#0#0#0#0#0#0#0#0#0#0#0#0#0#0#0\r\n0#0#0#0#0#0#0#1#0#0#0#0#0#0#0#0#0#0#0#0#0#0#0#1#0#0#0#0#0#0#0#1#0#0#0#0#0#0#0#0#0#0#0#0#0#0#0#1#0#0#0#0#0#0#0#0#0#0#0#0#0#0#0#0#0#0#0#0#0#0#0#0#0#0#0#0#0#0#0#0#0#0#0#0#0#0#0#0#0#0#0#0#0#0#0#0\r\n0#0#0#0#0#0#1#0#0#0#0#0#0#0#0#0#0#0#0#0#0#0#1#0#0#0#0#0#0#0#1#0#0#0#0#0#0#0#0#0#0#0#0#0#0#0#1#0#0#0#0#0#0#0#0#0#0#0#0#0#0#0#0#0#0#0#0#0#0#0#0#0#0#0#0#0#0#0#0#0#0#0#0#0#0#0#0#0#0#0#0#0#0#0#0#0\r\n0#0#0#0#0#1#0#0#0#0#0#0#0#0#0#0#0#0#0#0#0#1#0#0#0#0#0#0#0#1#0#0#0#0#0#0#0#0#0#0#0#0#0#0#0#1#0#0#0#0#0#0#0#0#0#0#0#0#0#0#0#0#0#0#0#0#0#0#0#0#0#0#0#0#0#0#0#0#0#0#0#0#0#0#0#0#0#0#0#0#0#0#0#0#0#0\r\n0#0#0#0#1#0#0#0#0#0#0#0#0#0#0#0#0#0#0#0#1#0#0#0#0#0#0#0#1#0#0#0#0#0#0#0#0#0#0#0#0#0#0#0#1#0#0#0#0#0#0#0#0#0#0#0#0#0#0#0#0#0#0#0#0#0#0#0#0#0#0#0#0#0#0#0#0#0#0#0#0#0#0#0#0#0#0#0#0#0#0#0#0#0#0#0\r\n0#0#0#1#0#0#0#0#0#0#0#0#0#0#0#0#0#0#0#1#0#0#0#0#0#0#0#1#0#0#0#0#0#0#0#0#0#0#0#0#0#0#0#1#0#0#0#0#0#0#0#0#0#0#0#0#0#0#0#0#0#0#0#0#0#0#0#0#0#0#0#0#0#0#0#0#0#0#0#0#0#0#0#0#0#0#0#0#0#0#0#0#0#0#0#0\r\n0#0#1#0#0#0#0#0#0#0#0#0#0#0#0#0#0#0#1#0#0#0#0#0#0#0#1#0#0#0#0#0#0#0#0#0#0#0#0#0#0#0#1#0#0#0#0#0#0#0#0#0#0#0#0#0#0#0#0#0#0#0#0#0#0#0#0#0#0#0#0#0#0#0#0#0#0#0#0#0#0#0#0#0#0#0#0#0#0#0#0#0#0#0#0#0\r\n0#1#0#0#0#0#0#0#0#0#0#0#0#0#0#0#0#1#0#0#0#0#0#0#0#1#0#0#0#0#0#0#0#0#0#0#0#0#0#0#0#1#0#0#0#0#0#0#0#0#0#0#0#0#0#0#0#0#0#0#0#0#0#0#0#0#0#0#0#0#0#0#0#0#0#0#0#0#0#0#0#0#0#0#0#0#0#0#0#0#0#0#0#0#0#0\r\n1#0#0#0#0#0#0#0#0#0#0#0#0#0#0#0#1#0#0#0#0#0#0#0#1#0#0#0#0#0#0#0#0#0#0#0#0#0#0#0#1#0#0#0#0#0#0#0#0#0#0#0#0#0#0#0#0#0#0#0#0#0#0#0#0#0#0#0#0#0#0#0#0#0#0#0#0#0#0#0#0#0#0#0#0#0#0#0#0#0#0#0#0#0#0#0\r\n0#0#0#0#0#0#0#1#0#0#0#0#0#0#0#0#0#0#0#0#0#0#0#1#0#0#0#0#0#0#0#1#0#0#0#0#0#0#0#0#0#0#0#0#0#0#0#1#0#0#0#0#0#0#0#0#0#0#0#0#0#0#0#0#0#0#0#0#0#0#0#0#0#0#0#0#0#0#0#0#0#0#0#0#0#0#0#0#0#0#0#0#0#0#0#0\r\n0#0#0#0#0#0#1#0#0#0#0#0#0#0#0#0#0#0#0#0#0#0#1#0#0#0#0#0#0#0#1#0#0#0#0#0#0#0#0#0#0#0#0#0#0#0#1#0#0#0#0#0#0#0#0#0#0#0#0#0#0#0#0#0#0#0#0#0#0#0#0#0#0#0#0#0#0#0#0#0#0#0#0#0#0#0#0#0#0#0#0#0#0#0#0#0\r\n0#0#0#0#0#1#0#0#0#0#0#0#0#0#0#0#0#0#0#0#0#1#0#0#0#0#0#0#0#1#0#0#0#0#0#0#0#0#0#0#0#0#0#0#0#1#0#0#0#0#0#0#0#0#0#0#0#0#0#0#0#0#0#0#0#0#0#0#0#0#0#0#0#0#0#0#0#0#0#0#0#0#0#0#0#0#0#0#0#0#0#0#0#0#0#0\r\n0#0#0#0#1#0#0#0#0#0#0#0#0#0#0#0#0#0#0#0#1#0#0#0#0#0#0#0#1#0#0#0#0#0#0#0#0#0#0#0#0#0#0#0#1#0#0#0#0#0#0#0#0#0#0#0#0#0#0#0#0#0#0#0#0#0#0#0#0#0#0#0#0#0#0#0#0#0#0#0#0#0#0#0#0#0#0#0#0#0#0#0#0#0#0#0\r\n0#0#0#1#0#0#0#0#0#0#0#0#0#0#0#0#0#0#0#1#0#0#0#0#0#0#0#1#0#0#0#0#0#0#0#0#0#0#0#0#0#0#0#1#0#0#0#0#0#0#0#0#0#0#0#0#0#0#0#0#0#0#0#0#0#0#0#0#0#0#0#0#0#0#0#0#0#0#0#0#0#0#0#0#0#0#0#0#0#0#0#0#0#0#0#0\r\n0#0#1#0#0#0#0#0#0#0#0#0#0#0#0#0#0#0#1#0#0#0#0#0#0#0#1#0#0#0#0#0#0#0#0#0#0#0#0#0#0#0#1#0#0#0#0#0#0#0#0#0#0#0#0#0#0#0#0#0#0#0#0#0#0#0#0#0#0#0#0#0#0#0#0#0#0#0#0#0#0#0#0#0#0#0#0#0#0#0#0#0#0#0#0#0\r\n0#1#0#0#0#0#0#0#0#0#0#0#0#0#0#0#0#1#0#0#0#0#0#0#0#1#0#0#0#0#0#0#0#0#0#0#0#0#0#0#0#1#0#0#0#0#0#0#0#0#0#0#0#0#0#0#0#0#0#0#0#0#0#0#0#0#0#0#0#0#0#0#0#0#0#0#0#0#0#0#0#0#0#0#0#0#0#0#0#0#0#0#0#0#0#0\r\n1#0#0#0#0#0#0#0#0#0#0#0#0#0#0#0#1#0#0#0#0#0#0#0#1#0#0#0#0#0#0#0#0#0#0#0#0#0#0#0#1#0#0#0#0#0#0#0#0#0#0#0#0#0#0#0#0#0#0#0#0#0#0#0#0#0#0#0#0#0#0#0#0#0#0#0#0#0#0#0#0#0#0#0#0#0#0#0#0#0#0#0#0#0#0#0\r\n0#0#0#0#0#1#0#0#0#0#0#0#0#0#0#0#0#0#0#0#0#1#0#0#0#0#0#0#0#0#0#1#0#0#0#0#0#0#0#0#0#0#0#0#0#0#0#0#0#0#0#0#0#0#0#0#0#0#0#0#0#0#0#0#0#0#0#0#0#0#0#0#0#0#0#0#0#0#0#0#0#0#0#0#0#0#0#0#0#0#0#0#0#0#0#0\r\n0#0#0#0#1#0#0#0#0#0#0#0#0#0#0#0#0#0#0#0#1#0#0#0#0#0#0#0#0#0#1#0#0#0#0#0#0#0#0#0#0#0#0#0#0#0#1#0#0#0#0#0#0#0#0#0#0#0#0#0#0#0#0#0#0#0#0#0#0#0#0#0#0#0#0#0#0#0#0#0#0#0#0#0#0#0#0#0#0#0#0#0#0#0#0#0\r\n0#0#0#1#0#0#0#0#0#0#0#0#0#0#0#0#0#0#0#1#0#0#0#0#0#1#0#0#0#0#0#0#0#0#0#0#0#0#0#0#0#1#0#0#0#0#0#0#0#0#0#0#0#0#0#0#0#0#0#0#0#0#0#0#0#0#0#0#0#0#0#0#0#0#0#0#0#0#0#0#0#0#0#0#0#0#0#0#0#0#0#0#0#0#0#0\r\n0#0#1#0#0#0#0#0#0#0#0#0#0#0#0#0#0#0#1#0#0#0#0#0#1#0#0#0#0#0#0#0#0#0#0#0#0#0#0#0#1#0#0#0#0#0#0#0#0#0#0#0#0#0#0#0#0#0#0#0#0#0#0#0#0#0#0#0#0#0#0#0#0#0#0#0#0#0#0#0#0#0#0#0#0#0#0#0#0#0#0#0#0#0#0#0\r\n0#0#0#0#0#0#0#0#0#0#0#0#0#0#0#0#0#0#0#0#0#0#0#0#0#0#0#0#0#0#0#0#0#0#0#0#0#0#0#0#0#0#0#0#0#0#0#0#0#0#0#0#0#0#0#0#0#0#0#0#0#0#0#0#0#0#0#0#0#0#0#0#0#0#0#0#0#0#0#0#0#0#0#0#0#0#0#0#0#0#0#0#0#0#0#0\r\n0#0#0#0#0#0#0#0#0#0#0#0#0#0#0#0#0#0#0#0#0#0#0#0#0#0#0#0#0#0#0#0#0#0#0#0#0#0#0#0#0#0#0#0#0#0#0#0#0#0#0#0#0#0#0#0#0#0#0#0#0#0#0#0#0#0#0#0#0#0#0#0#0#0#0#0#0#0#0#0#0#0#0#0#0#0#0#0#0#0#0#0#0#0#0#0\r\n0#0#0#0#0#0#0#0#0#0#0#0#0#0#0#0#0#0#0#0#0#0#0#0#0#0#0#0#0#0#0#0#0#0#0#0#0#0#0#0#0#0#0#0#0#0#0#0#0#0#0#0#0#0#0#0#0#0#0#0#0#0#0#0#0#0#0#0#0#0#0#0#0#0#0#0#0#0#0#0#0#0#0#0#0#0#0#0#0#0#0#0#0#0#0#0\r\n0#0#0#0#0#0#0#0#0#0#0#0#0#0#0#0#0#0#0#0#0#0#0#0#0#0#0#0#0#0#0#0#0#0#0#0#0#0#0#0#0#0#0#0#0#0#0#0#0#0#0#0#0#0#0#0#0#0#0#0#0#0#0#0#0#0#0#0#0#0#0#0#0#0#0#0#0#0#0#0#0#0#0#0#0#0#0#0#0#0#0#0#0#0#0#0\r\n0#0#0#0#0#0#0#0#0#0#0#0#0#0#0#0#0#0#0#0#0#0#0#0#0#0#0#0#0#0#0#0#0#0#0#0#0#0#0#0#0#0#0#0#0#0#0#0#0#0#0#0#0#0#0#0#0#0#0#0#0#0#0#0#0#0#0#0#0#0#0#0#0#0#0#0#0#0#0#0#0#0#0#0#0#0#0#0#0#0#0#0#0#0#0#0\r\n0#0#0#0#0#0#0#0#0#0#0#0#0#0#0#0#0#0#0#0#0#0#0#0#0#0#0#0#0#0#0#0#0#0#0#0#0#0#0#0#0#0#0#0#0#0#0#0#0#0#0#0#0#0#0#0#0#0#0#0#0#0#0#0#0#0#0#0#0#0#0#0#0#0#0#0#0#0#0#0#0#0#0#0#0#0#0#0#0#0#0#0#0#0#0#0\r\n0#0#0#0#0#0#0#0#0#0#0#0#0#0#0#0#0#0#0#0#0#0#0#0#0#0#0#0#0#0#0#0#0#0#0#0#0#0#0#0#0#0#0#0#0#0#0#0#0#0#0#0#0#0#0#0#0#0#0#0#0#0#0#0#0#0#0#0#0#0#0#0#0#0#0#0#0#0#0#0#0#0#0#0#0#0#0#0#0#0#0#0#0#0#0#0\r\n0#0#0#0#0#0#0#0#0#0#0#0#0#0#0#0#0#0#0#0#0#0#0#0#0#0#0#0#0#0#0#0#0#0#0#0#0#0#0#0#0#0#0#0#0#0#0#0#0#0#0#0#0#0#0#0#0#0#0#0#0#0#0#0#0#0#0#0#0#0#0#0#0#0#0#0#0#0#0#0#0#0#0#0#0#0#0#0#0#0#0#0#0#0#0#0\r\n0#0#0#0#0#0#0#0#0#0#0#0#0#0#0#0#0#0#0#0#0#0#0#0#0#0#0#0#0#0#0#0#0#0#0#0#0#0#0#0#0#0#0#0#0#0#0#0#0#0#0#0#0#0#0#0#0#0#0#0#0#0#0#0#0#0#0#0#0#0#0#0#0#0#0#0#0#0#0#0#0#0#0#0#0#0#0#0#0#0#0#0#0#0#0#0\r\n0#0#0#0#0#0#0#0#0#0#0#0#0#0#0#0#0#0#0#0#0#0#0#0#0#0#0#0#0#0#0#0#0#0#0#0#0#0#0#0#0#0#0#0#0#0#0#0#0#0#0#0#0#0#0#0#0#0#0#0#0#0#0#0#0#0#0#0#0#0#0#0#0#0#0#0#0#0#0#0#0#0#0#0#0#0#0#0#0#0#0#0#0#0#0#0\r\n0#0#0#0#0#0#0#0#0#0#0#0#0#0#0#0#0#0#0#0#0#0#0#0#0#0#0#0#0#0#0#0#0#0#0#0#0#0#0#0#0#0#0#0#0#0#0#0#0#0#0#0#0#0#0#0#0#0#0#0#0#0#0#0#0#0#0#0#0#0#0#0#0#0#0#0#0#0#0#0#0#0#0#0#0#0#0#0#0#0#0#0#0#0#0#0\r\n0#0#0#0#0#0#0#0#0#0#0#0#0#0#0#0#0#0#0#0#0#0#0#0#0#0#0#0#0#0#0#0#0#0#0#0#0#0#0#0#0#0#0#0#0#0#0#0#0#0#0#0#0#0#0#0#0#0#0#0#0#0#0#0#0#0#0#0#0#0#0#0#0#0#0#0#0#0#0#0#0#0#0#0#0#0#0#0#0#0#0#0#0#0#0#0\r\n0#0#0#0#0#0#0#0#0#0#0#0#0#0#0#0#0#0#0#0#0#0#0#0#0#0#0#0#0#0#0#0#0#0#0#0#0#0#0#0#0#0#0#0#0#0#0#0#0#0#0#0#0#0#0#0#0#0#0#0#0#0#0#0#0#0#0#0#0#0#0#0#0#0#0#0#0#0#0#0#0#0#0#0#0#0#0#0#0#0#0#0#0#0#0#0\r\n0#0#0#0#0#0#0#0#0#0#0#0#0#0#0#0#0#0#0#0#0#0#0#0#0#0#0#0#0#0#0#0#0#0#0#0#0#0#0#0#0#0#0#0#0#0#0#0#0#0#0#0#0#0#0#0#0#0#0#0#0#0#0#0#0#0#0#0#0#0#0#0#0#0#0#0#0#0#0#0#0#0#0#0#0#0#0#0#0#0#0#0#0#0#0#0\r\n0#0#0#0#0#0#0#0#0#0#0#0#0#0#0#0#0#0#0#0#0#0#0#0#0#0#0#0#0#0#0#0#0#0#0#0#0#0#0#0#0#0#0#0#0#0#0#0#0#0#0#0#0#0#0#0#0#0#0#0#0#0#0#0#0#0#0#0#0#0#0#0#0#0#0#0#0#0#0#0#0#0#0#0#0#0#0#0#0#0#0#0#0#0#0#0\r\n0#0#0#0#0#0#0#0#0#0#0#0#0#0#0#0#0#0#0#0#0#0#0#0#0#0#0#0#0#0#0#0#0#0#0#0#0#0#0#0#0#0#0#0#0#0#0#0#0#0#0#0#0#0#0#0#0#0#0#0#0#0#0#0#0#0#0#0#0#0#0#0#0#0#0#0#0#0#0#0#0#0#0#0#0#0#0#0#0#0#0#0#0#0#0#0\r\n0#0#0#0#0#0#0#0#0#0#0#0#0#0#0#0#0#0#0#0#0#0#0#0#0#0#0#0#0#0#0#0#0#0#0#0#0#0#0#0#0#0#0#0#0#0#0#0#0#0#0#0#0#0#0#0#0#0#0#0#0#0#0#0#0#0#0#0#0#0#0#0#0#0#0#0#0#0#0#0#0#0#0#0#0#0#0#0#0#0#0#0#0#0#0#0\r\n0#0#0#0#0#0#0#0#0#0#0#0#0#0#0#0#0#0#0#0#0#0#0#0#0#0#0#0#0#0#0#0#0#0#0#0#0#0#0#0#0#0#0#0#0#0#0#0#0#0#0#0#0#0#0#0#0#0#0#0#0#0#0#0#0#0#0#0#0#0#0#0#0#0#0#0#0#0#0#0#0#0#0#0#0#0#0#0#0#0#0#0#0#0#0#0\r\n0#0#0#0#0#0#0#0#0#0#0#0#0#0#0#0#0#0#0#0#0#0#0#0#0#0#0#0#0#0#0#0#0#0#0#0#0#0#0#0#0#0#0#0#0#0#0#0#0#0#0#0#0#0#0#0#0#0#0#0#0#0#0#0#0#0#0#0#0#0#0#0#0#0#0#0#0#0#0#0#0#0#0#0#0#0#0#0#0#0#0#0#0#0#0#0\r\n", "0", "", "0", "", ""]
  out "Project Information":string="TX1#TX1-RX1#TX2-RX1#SDD21##TDD11#1#D:\\CALFILES\\#D:\\HPTS Development\\VNA Automatic Data Save Tool 20150708\\Templete\\QSFP+_IBM New.xlsx#0#0.000000\r\nRX1#TX2-RX1#TX3-RX1#SDD22##TDD22#2##TDD11\t1\t2\t0@TDD22\t2\t2\t0@SDD21\t3\t2\t0@SDD22\t4\t2\t0@SCD21\t5\t2\t0@SCD22\t6\t2\t0@SCC11\t7\t2\t0@NEXT\t8\t2\t0@FEXT\t9\t2\t0@##5.000000\r\nTX2#TX3-RX1#TX4-RX1#SCD21###3##Applicant\t0\t2\t1@Part Name\t0\t3\t1@Part Number\t0\t4\t1@Report No\t0\t2\t12@Sample No\t0\t4\t12@Prepared By\t0\t63\t0@Approved By\t0\t63\t6@Date\t0\t63\t2@Thru Result\t0\t13\t5@##4000\r\nRX2#TX4-RX1#TX1-RX2#SCD22###4####50.000000\r\nTX3#TX1-RX2#TX3-RX2#SCC11###5####-2.000000\r\nRX3#TX2-RX2#TX4-RX2#NEXT###6####1\r\nTX4#TX3-RX2#TX1-RX3#FEXT###7####1@110@2@105;1@90@2@95\r\nRX4#TX4-RX2#TX2-RX3########0.000\r\n#TX1-RX3#TX4-RX3########10.0\r\n#TX2-RX3#TX1-RX4########\r\n#TX3-RX3#TX2-RX4########\r\n#TX4-RX3#TX3-RX4########\r\n#TX1-RX4#########\r\n#TX2-RX4#########\r\n#TX3-RX4#########\r\n#TX4-RX4#########\r\n"
